vi "Launcher.vi"   [LabVIEW 2023]
doc: "Launch the top-level coffee shop Actor."
uses:
  Classes/Coffee Shop/Coffee Shop.lvclass
  c:/dev/_r/4/eng/lv-core/lvpostprocessingd/lv_mc_x86_64/dist_i386/vi.lib/ActorFramework/Actor/Actor.lvclass
  <vilib>/ActorFramework/Actor/Actor.lvclass
panel:
  # "Overview: Demonstrates the use of the Actor Framework to create a simulation of a coffee shop.  This simulation is based on the interaction model described in this article: http://www.eaipatterns.com/docs/IEEE_Software_Design_2PC.pdf\n\nInstructions:\n1. Run this VI to launch the main coffee shop actor.  This VI will close once the coffee shop is launched.\n2.  Refer to the front panel of the coffee shop actor for instructions on how to interact with the coffee shop.\n3.  For more details on the design choices made in this simulation, refer to the ReadMe.html document provided in the project."
  # "Launching Coffee Shop..."
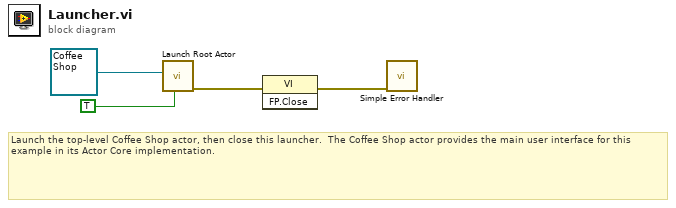
[diagram p0: block diagram]
diagram:
  # "Launch the top-level Coffee Shop actor, then close this launcher.  The Coffee Shop actor provides the main user interface for this example in its Actor Core implementation."
  n1 = call <vilib>:"Launch Root Actor.vi"("Open Actor Core front panel? (F)"=TRUE, "Actor"=refnum<class "Coffee Shop.lvclass"> refnum ("Coffee Shop.lvclass")) -> ("error out"=w2:errorcluster)  [unwired: 8 in, 1 out]
  n2 = invoke class="VI" method="FP.Close"(error in=w2) -> (error out=w1:errorcluster)  [unwired: 2 in, 2 out]
  n3 = call <vilib>:"Simple Error Handler.vi"("error in (no error)"=w1) -> ()  [unwired: 4 in, 5 out]
